vi "Joystick 2 Ball Intake System.vi"(8 "Drive Joystick Values":dbl[](array[numeric]), 9 "Secondary Joystick Values":dbl[](array[numeric]), 10 "Drive Joystick Buttons":bool[](array[boolean]), 11 "Secondary Joystick Buttons":bool[](array[boolean])) -> (0 "Ball System Actions":T1)   [LabVIEW 2019]
uses:
  Controls/Ball System Actions.ctl
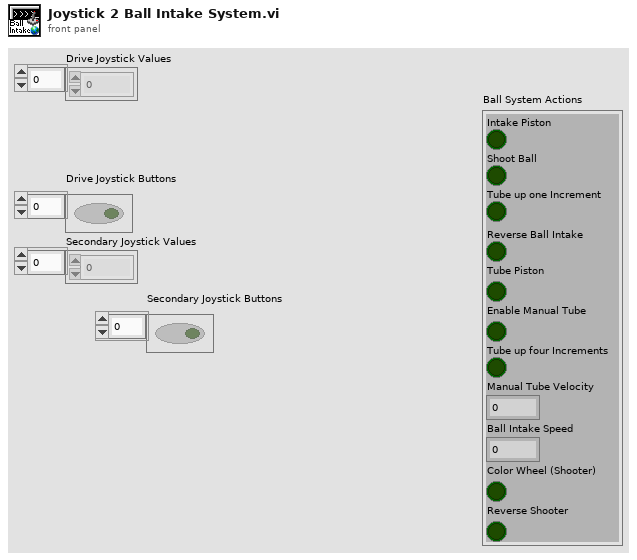
[diagram p1: front panel]
types:
  T1 = typedef "Ball System Actions.ctl" = cluster{"Intake Piston ":bool, "Shoot Ball":bool, "Tube up one Increment\t":bool, "Reverse Ball Intake":bool, "Tube Piston":bool, "Enable Manual Tube":bool, "Tube up four Increments":bool, "Manual Tube Velocity":dbl, "Ball Intake Speed":dbl, "Color Wheel (Shooter)":bool, "Reverse Shooter":bool}
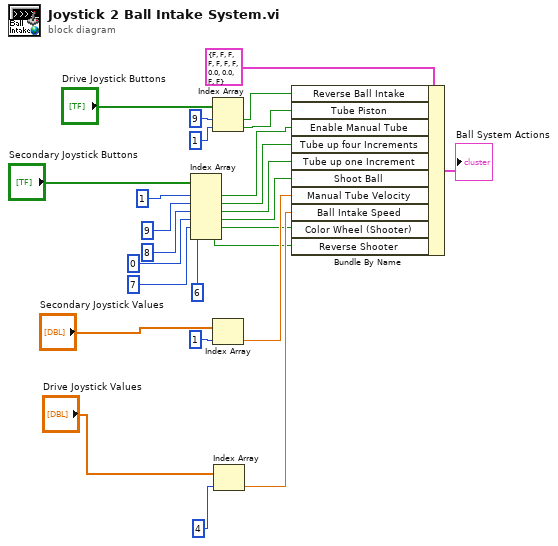
[diagram p0: block diagram]
diagram:
  n1 = Index Array(array="Secondary Joystick Buttons", index #1=1 ("index"), index #2=9 ("index"), index #3=8 ("index"), index #4=0 ("index"), index #5=7 ("index"), index #6=6 ("index")) -> (element #1=w7:bool, element #2=w18:bool, element #3=w17:bool, element #4=w15:bool, element #5=w3:bool, element #6=w1:bool)
  n2 = Index Array(array="Drive Joystick Buttons", index #1=9 ("index"), index #2=1 ("index")) -> (element #1=w19:bool, element #2=w9:bool)
  n3 = Index Array(array="Secondary Joystick Values", index=1) -> (element=w13:dbl)
  n4 = Index Array(array="Drive Joystick Values", index=4) -> (element=w5:dbl)
  n5 = Bundle By Name(cluster=T1 {"Intake Piston "=FALSE, "Shoot Ball"=FALSE, "Tube up one Increment\t"=FALSE, "Reverse Ball Intake"=FALSE, "Tube Piston"=FALSE, "Enable Manual Tube"=FALSE, "Tube up four Increments"=FALSE, "Manual Tube Velocity"=0.0, "Ball Intake Speed"=0.0, "Color Wheel (Shooter)"=FALSE, "Reverse Shooter"=FALSE} ("Ball System Actions"), "Reverse Ball Intake"=w19, "Tube Piston"=w9, "Enable Manual Tube"=w7, "Tube up four Increments"=w18, "Tube up one Increment"=w17, "Shoot Ball"=w15, "Manual Tube Velocity"=w13, "Ball Intake Speed"=w5, "Color Wheel (Shooter)"=w3, "Reverse Shooter"=w1) -> (→"Ball System Actions":T1)
